vi "Change Mode.vi"(8 "error in":errorcluster, 10 "Change Mode Cluster":T1, 11 "Message Handling Cluster in":T2) -> (0 "error out":errorcluster, 3 "Message Handling Cluster out":T2)   [LabVIEW 2024]
uses:
  Controls/Clusters/Message Handling Cluster.ctl
  Controls/Clusters/Change Mode Cluster.ctl
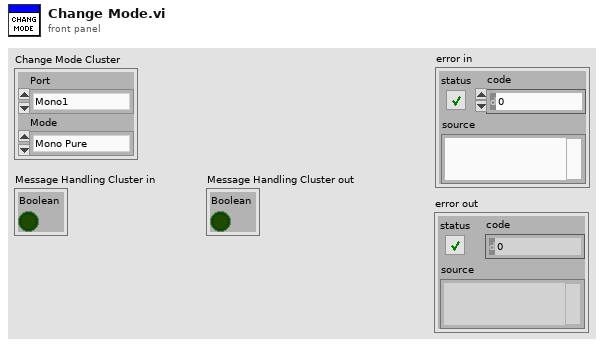
[diagram p1: front panel]
types:
  T1 = typedef "Change Mode Cluster.ctl" = cluster{"Port":enum16{"Mono1", "Mono2", "Bipolar", "Ligasure"}, "Mode":enum16{"Mono Pure", "Mono Blend", "Mono Fulgerate", "Mono Spray", "Bi Precision", "Bi Macro", "Bi Standard"}}
  T2 = typedef "Message Handling Cluster.ctl" = cluster{"Boolean":bool}
  T3 = enum16{"Mono Pure", "Mono Blend", "Mono Fulgerate", "Mono Spray", "Bi Precision", "Bi Macro", "Bi Standard"}
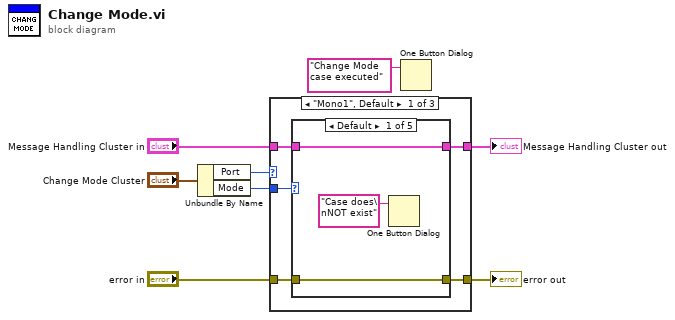
[diagram p0: block diagram]
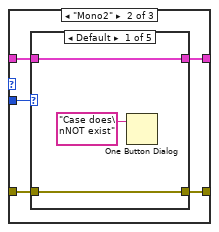
[diagram p6: hidden frame]
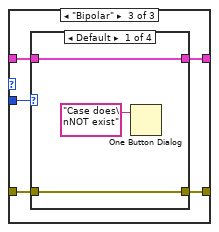
[diagram p11: hidden frame]
diagram:
  n1 = Unbundle By Name("Change Mode Cluster") -> ("Port"=w4:enum16{"Mono1", "Mono2", "Bipolar", "Ligasure"}, "Mode"=w1:T3)
  n2 = case shown="\"Mono1\", Default" w4 {
    tunnel: "Message Handling Cluster in" -> [w9 w25 w41]
    tunnel: [w10 w26 w42] -> w8
    tunnel: [w13 w29 w45] -> w3
    tunnel: "error in" -> [w12 w28 w44]
    tunnel: w1 -> [w11 w27 w43]
    frame "Mono1", Default {
      n3 = case shown="Default" w11 {
        tunnel: [w16 w18 w20 w22 w24] -> w13
        tunnel: w12 -> [w16 w18 w20 w22 w24]
        tunnel: [w15 w17 w19 w21 w23] -> w10
        tunnel: w9 -> [w15 w17 w19 w21 w23]
        frame Default {
          n4 = One Button Dialog(message="Case does\nNOT exist") -> ()  [unwired: 1 in, 1 out]
        }
        frame "Mono Pure" {
        }
        frame "Mono Blend" {
        }
        frame "Mono Fulgerate" {
        }
        frame "Mono Spray" {
        }
      }
    }
    frame "Mono2" {
      n5 = case shown="Default" w27 {
        tunnel: [w32 w34 w36 w38 w40] -> w29
        tunnel: w28 -> [w32 w34 w36 w38 w40]
        tunnel: [w31 w33 w35 w37 w39] -> w26
        tunnel: w25 -> [w31 w33 w35 w37 w39]
        frame Default {
          n6 = One Button Dialog(message="Case does\nNOT exist") -> ()  [unwired: 1 in, 1 out]
        }
        frame "Mono Pure" {
        }
        frame "Mono Blend" {
        }
        frame "Mono Fulgerate" {
        }
        frame "Mono Spray" {
        }
      }
    }
    frame "Bipolar" {
      n7 = case shown="Default" w43 {
        tunnel: [w48 w50 w52 w54] -> w45
        tunnel: w44 -> [w48 w50 w52 w54]
        tunnel: [w47 w49 w51 w53] -> w42
        tunnel: w41 -> [w47 w49 w51 w53]
        frame Default {
          n8 = One Button Dialog(message="Case does\nNOT exist") -> ()  [unwired: 1 in, 1 out]
        }
        frame "Bi Precision" {
        }
        frame "Bi Macro" {
        }
        frame "Bi Standard" {
        }
      }
    }
  }
  "Message Handling Cluster out" <- w8
  "error out" <- w3
  n9 = One Button Dialog(message="Change Mode case executed") -> ()  [unwired: 1 in, 1 out]
